vi "Transfer Group Errors.vi"   [LabVIEW 2017, in "Data Sharing Framework Core.lvlib" / "Data Sharing Framework Engine.lvlib" / "Transfer Group.lvclass"]
uses:
  Transfer Group.lvclass
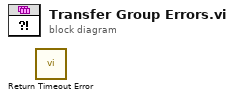
[diagram p0: block diagram]
diagram:
  n1 = call "Return Timeout Error.vi"() -> ()  [unwired: 10 in, 2 out]
